vi "Out of Bounds.vi"(8 "Percent / Fixed":bool, 9 "+/-":dbl, 10 "Nominal":dbl, 11 "Measured Value":dbl) -> (2 "Out of Bounds":bool)   [LabVIEW 2019]
doc: "This VI returns TRUE if the \"Measured Value\" input is outside of the bounds calcualted by the \"Nomial\" and \"+/-\" inputs.\n\nIf the \"Percent/Fixed\" Input is TRUE than the \"+/-\" value is used as a percentage of the \"Nominal\" to calculate the tolerance limits\n\nIf the \"Percent/Fixed\" Input is FALSE than he \"+/-\" value is used as a fixed tolerance to calculate the tolerance limits"
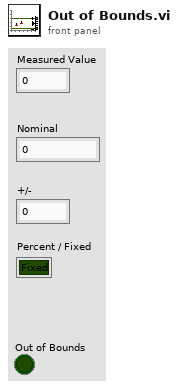
[diagram p1: front panel]
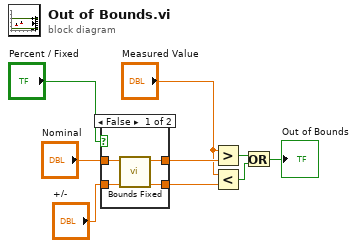
[diagram p0: block diagram]
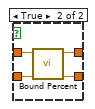
[diagram p2: hidden frame]
diagram:
  n1 = case shown="False" "Percent / Fixed" {
    tunnel: "+/-" -> [w12 w17]
    tunnel: "Nominal" -> [w13 w16]
    tunnel: [w11 w15] -> w6
    tunnel: [w10 w14] -> w1
    frame False {
      n2 = call <userlib>:"Bounds Fixed.vi"("+/-"=w12, "Nominal"=w13) -> ("Min"=w10:dbl, "Max"=w11:dbl)  [unwired: 8 in]
    }
    frame True {
      n3 = call <userlib>:"Bound Percent.vi"("Tolerance %"=w17, "Nominal"=w16) -> ("Min"=w14:dbl, "Max"=w15:dbl)  [unwired: 8 in]
    }
  }
  n4 = Greater?(x="Measured Value", y=w6) -> (0:w5:bool)
  n5 = Less?(x="Measured Value", y=w1) -> (x < y?=w4:bool)
  n6 = Or(x=w5, y=w4) -> (x .or. y?=→"Out of Bounds":bool)
